vi "Save Samples.vi"(6 "Type of Feature":string, 8 "error in (no error)":errorcluster, 10 "Image":T1, 11 "Destination Folder":path) -> (0 "error out":errorcluster)   [LabVIEW 2013]
uses:
  <vilib>/vision/Image Controls.llb/IMAQ Image.ctl
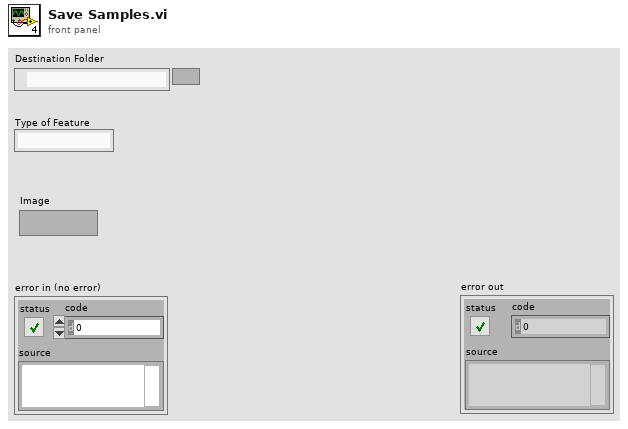
[diagram p1: front panel]
types:
  T1 = typedef "IMAQ Image.ctl" = refnum<image>
  T2 = enum16{"open", "replace", "create", "open or create", "replace or create", "replace or create with confirmation"}
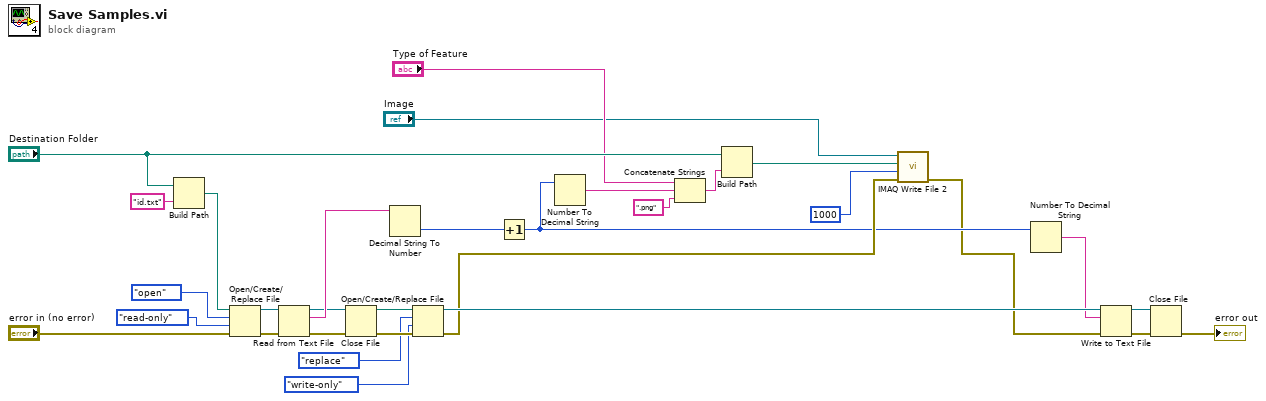
[diagram p0: block diagram]
diagram:
  n1 = Build Path(base path="Destination Folder", name or relative path="id.txt") -> (appended path=w31:path)
  n2 = Open/Create/Replace File(file path (use dialog)=w31, error in="error in (no error)", operation (0:open)=T2."open", access (0:read/write)=enum16{"read/write", "read-only", "write-only"}."read-only") -> (refnum out=w30:refnum<file>, error out=w29:errorcluster)  [unwired: 2 in, 1 out]
  n3 = Read from Text File(file (use dialog)=w30, error in=w29) -> (refnum out=w21:refnum<file>, text=w28:string, error out=w22:errorcluster)  [unwired: 2 in, 1 out]
  n4 = Close File(refnum=w21, error in=w22) -> (path=w19:path, error out=w20:errorcluster)
  n5 = Decimal String To Number(string=w28) -> (number=w27:i32)  [unwired: 2 in, 1 out]
  n6 = Open/Create/Replace File(file path (use dialog)=w19, error in=w20, operation (0:open)=T2."replace", access (0:read/write)=enum16{"read/write", "read-only", "write-only"}."write-only") -> (refnum out=w16:refnum<file>, error out=w9:errorcluster)  [unwired: 2 in, 1 out]
  n7 = Increment(x=w27) -> (x+1=w8:i32)
  n8 = Number To Decimal String(number=w8) -> (decimal integer string=w5:string)  [unwired: 1 in]
  n9 = Concatenate Strings("Type of Feature", w5, ".png" ("string")) -> (w3:string)
  n10 = Build Path(base path="Destination Folder", name or relative path=w3) -> (appended path=w2:path)
  n11 = call-poly "IMAQ Write File 2"("error in (no error)"=w9, "Image Quality"=u32 1000, "File Path"=w2, "Image"="Image") -> ("error out"=w7:errorcluster)  [unwired: 6 in, 1 out]
  n12 = Number To Decimal String(number=w8) -> (decimal integer string=w6:string)  [unwired: 1 in]
  n13 = Write to Text File(file (use dialog)=w16, text=w6, error in=w7) -> (refnum out=w24:refnum<file>, error out=w23:errorcluster)  [unwired: 1 in, 1 out]
  n14 = Close File(refnum=w24, error in=w23) -> (error out=→"error out":errorcluster)  [unwired: 1 out]
